vi "ConfigCreateProgram.vi"(9 "Positions":string[][](array[string]), 10 "Microscope":string[][](array[string]), 11 "Single Feed Cycle Refresh Ratio":dbl[](array[numeric])) -> (2 "ProgramPath":path, 3 "ProgramStopped":bool)   [LabVIEW 2018, in "Config.lvlib"]
uses:
  Config.lvlib
  <vilib>/Analysis/baseanly.llb/Mean (DBL).vi
  <vilib>/xml/Load XML File.vi
  <vilib>/xml/Close Reference(Node).vi
  <vilib>/xml/NI_XML.lvlib
  <vilib>/Analysis/NI_AALBase.lvlib
panel:
  out "LoopEndNumber":u16
  out "LoopStartNumber":u16
  in  "error in":errorcluster
  in  "Calc Minimal Acqu time":bool
  out "Minimal Acquisition Time":dbl format="%<%H:%M:%S>t"
  out "Micro Ok?":bool
  in  "Microscope Settings":path
  out "Pos Ok?":bool
  in  "Load Positions":path
  in  "Acquire":bool
  in  "Loop End":bool
  in  "Loop Start":bool
  in  "Incubate":bool
  in  "Change Reagent":bool
  in  "Feed":bool
  in  "Mix":bool
  out "error out":errorcluster
  in  "Program Steps":i32(listbox)
  in  "stop":bool
  in  "Load old Prog":bool
  in  "Clear":bool
  in  "Save":bool
  # "Program Creation"
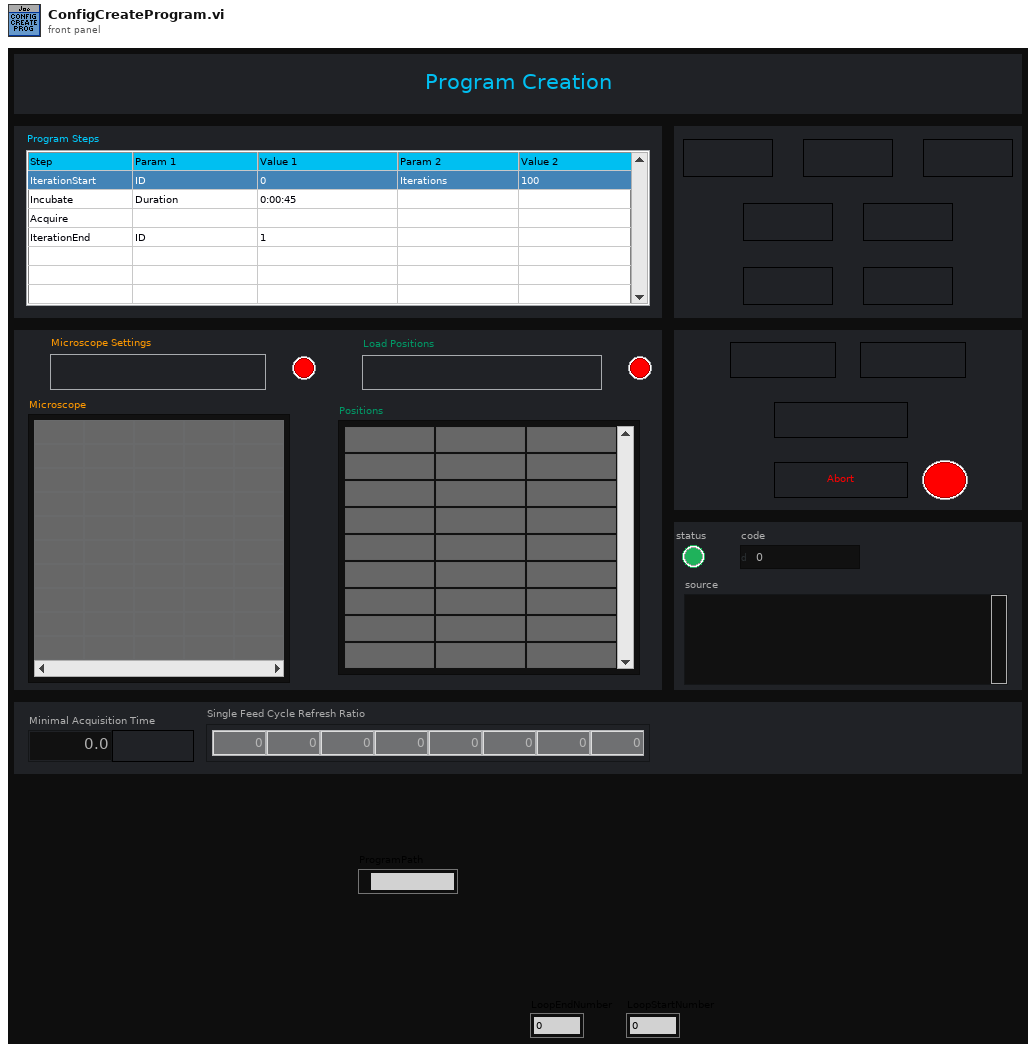
[diagram p1: front panel]
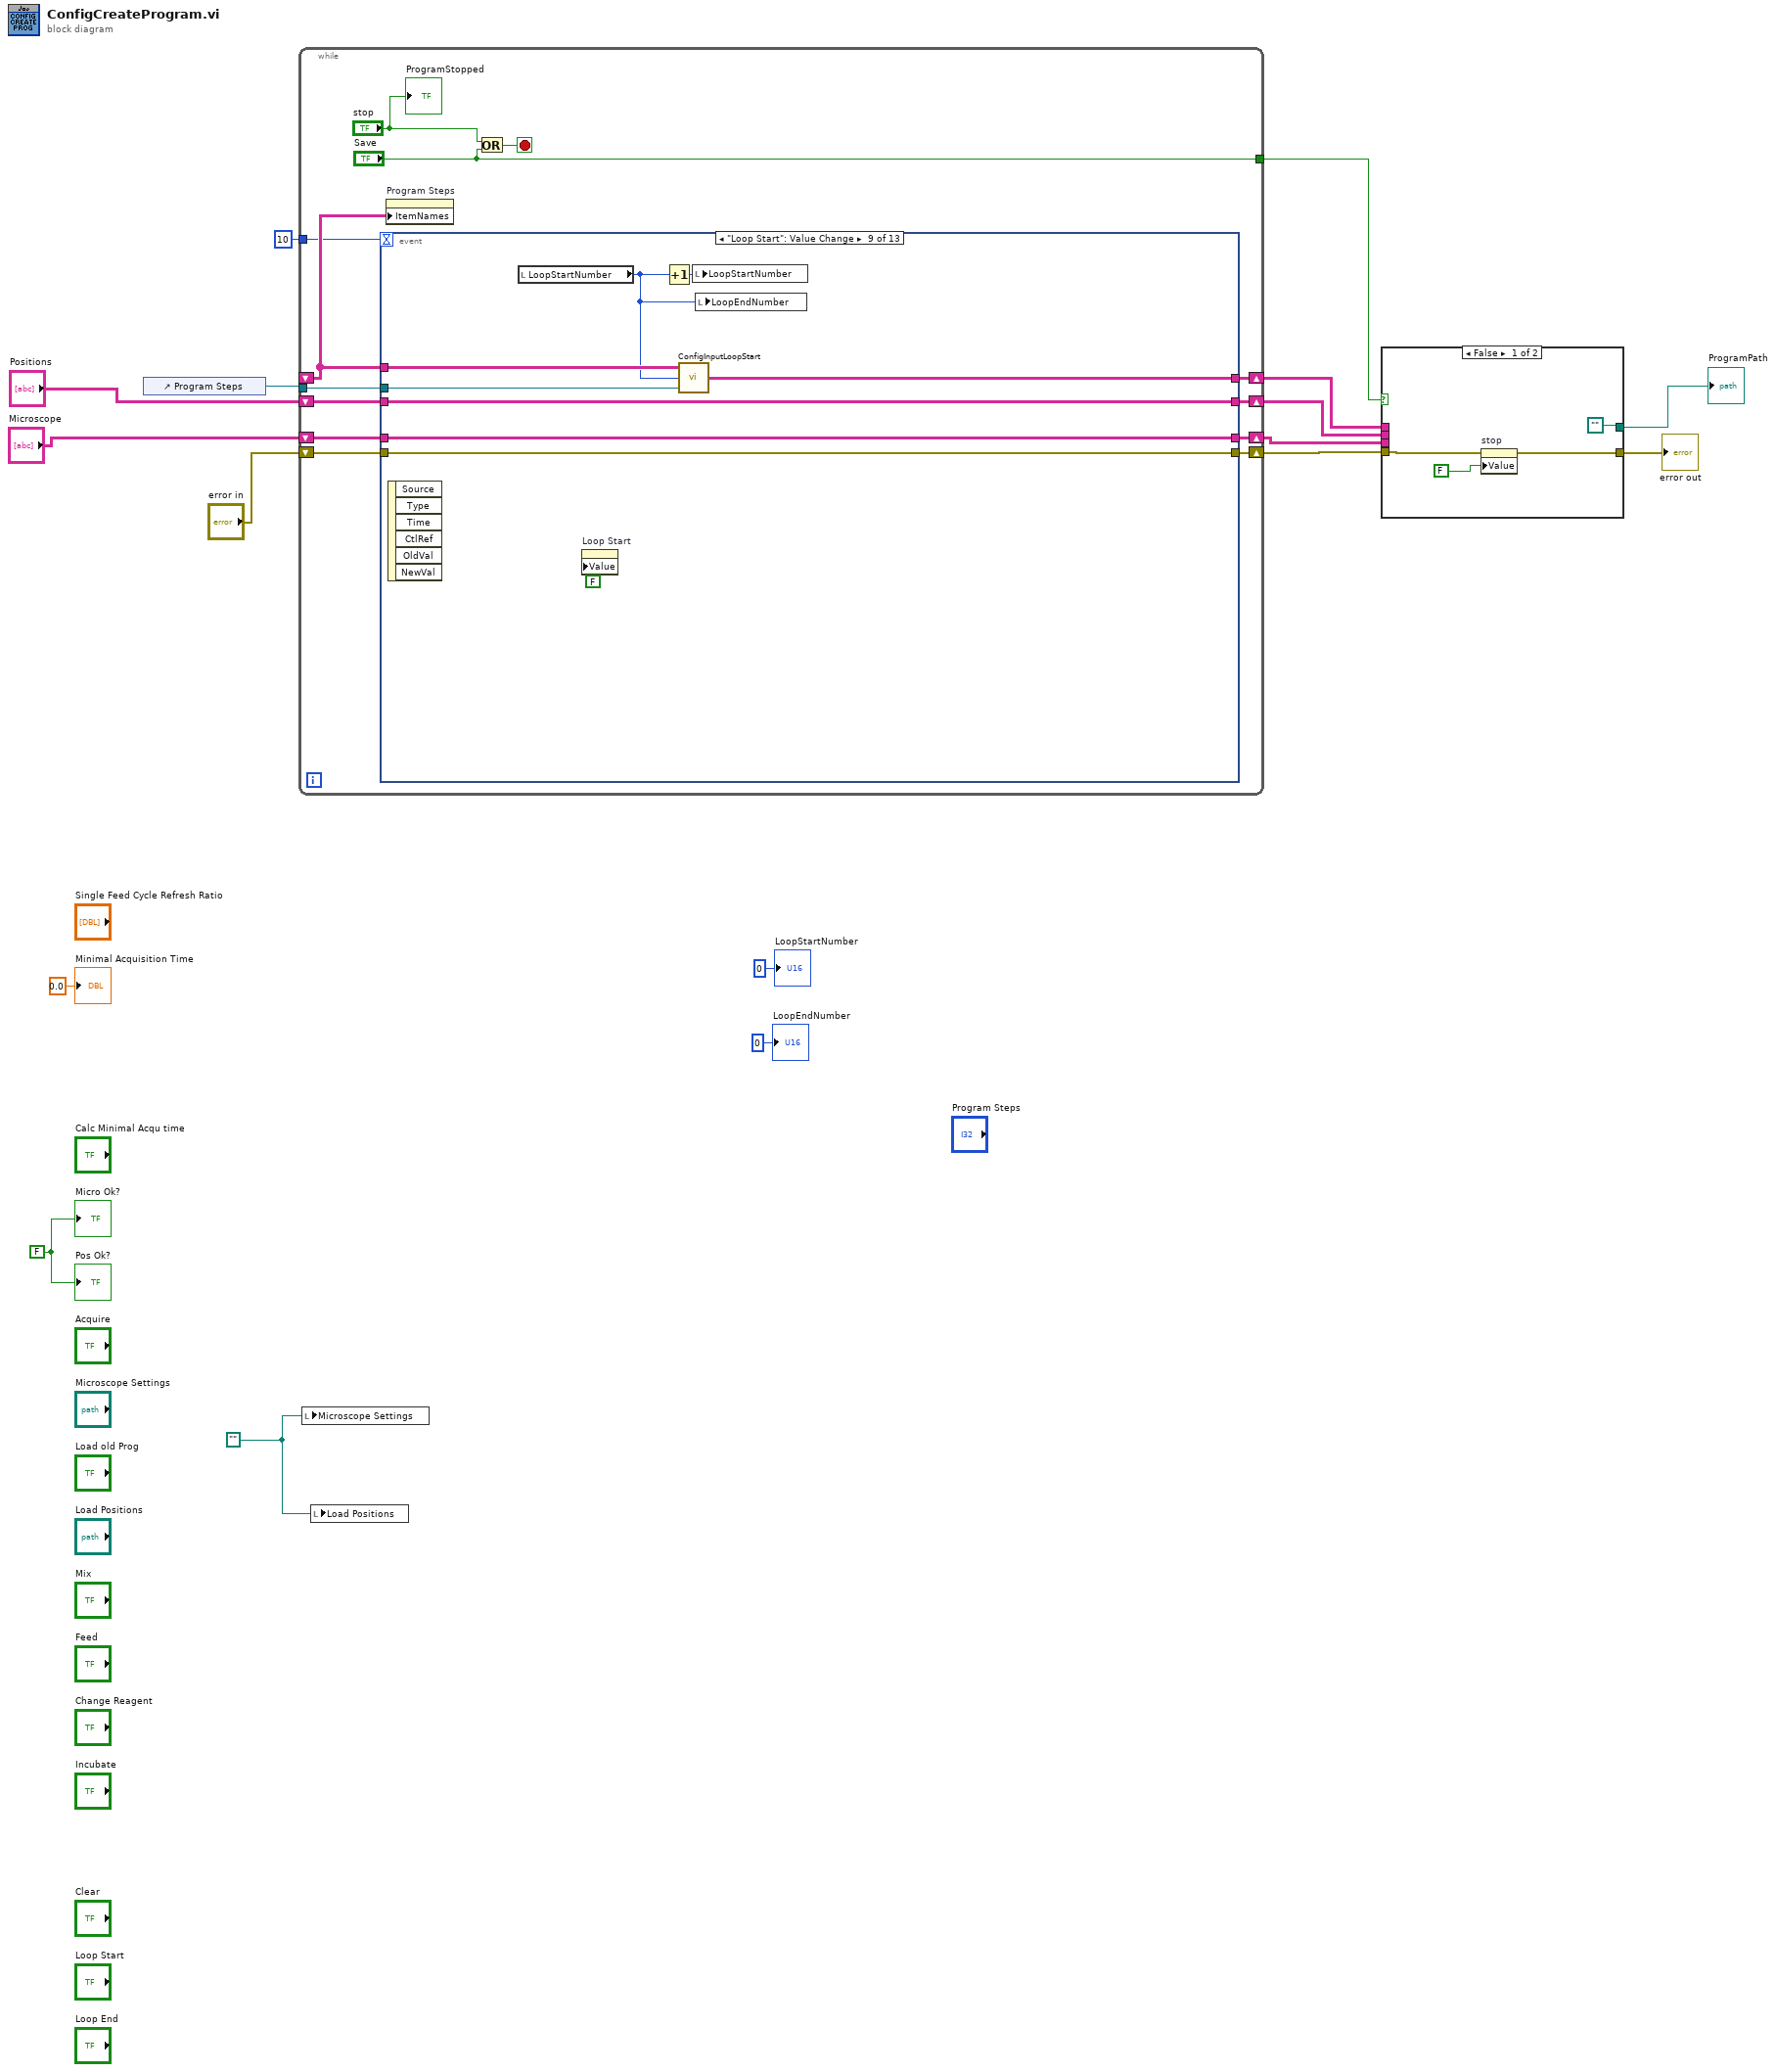
[diagram p0: block diagram]
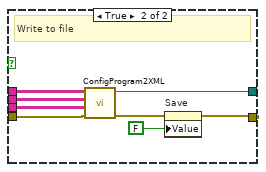
[diagram p2: hidden frame]
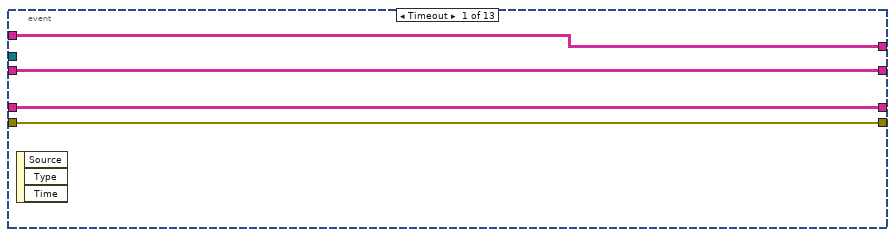
[diagram p3: hidden frame]
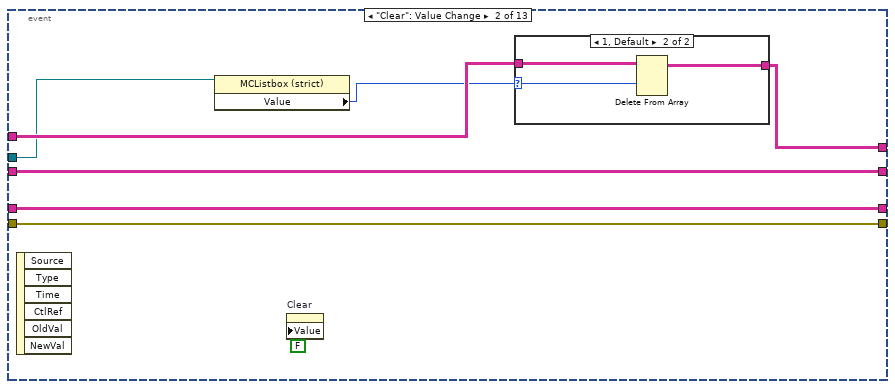
[diagram p4: hidden frame]
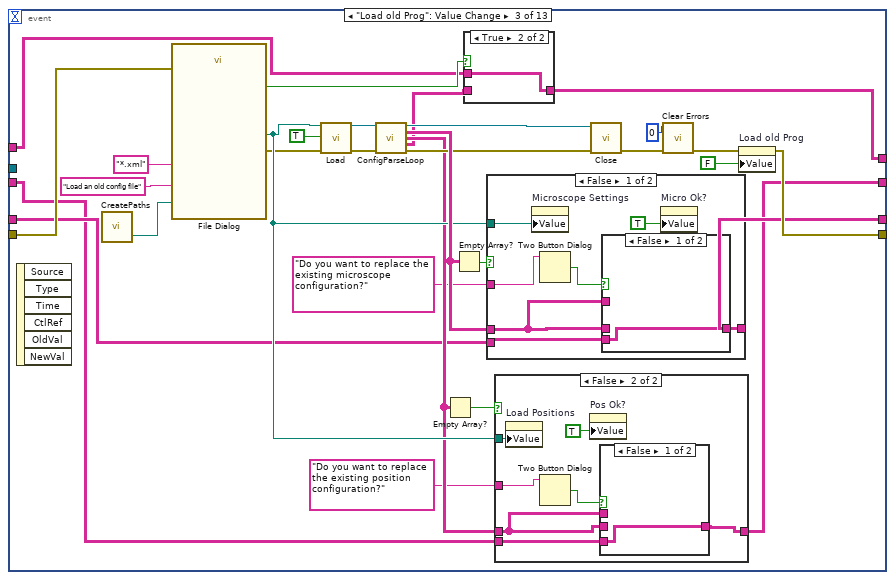
[diagram p6: hidden frame]
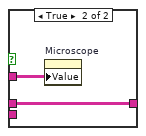
[diagram p8: hidden frame]
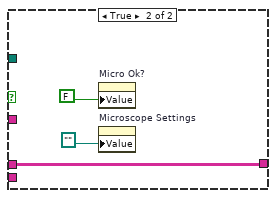
[diagram p9: hidden frame]
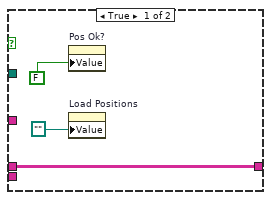
[diagram p10: hidden frame]
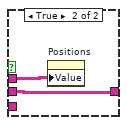
[diagram p11: hidden frame]
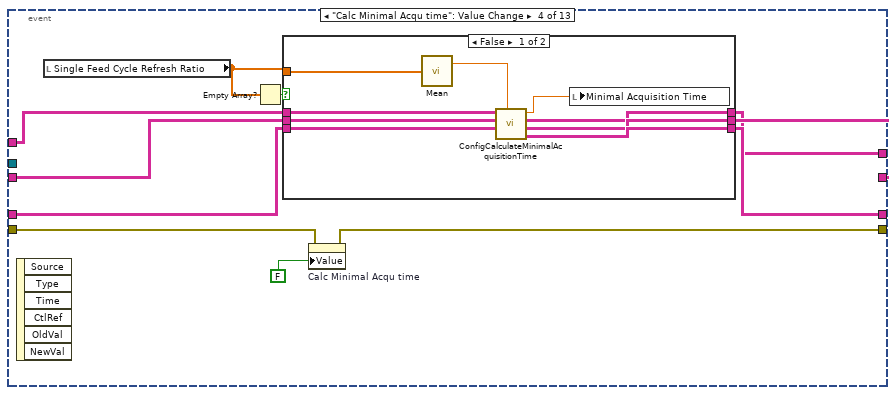
[diagram p12: hidden frame]
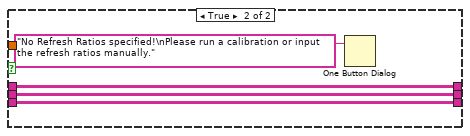
[diagram p13: hidden frame]
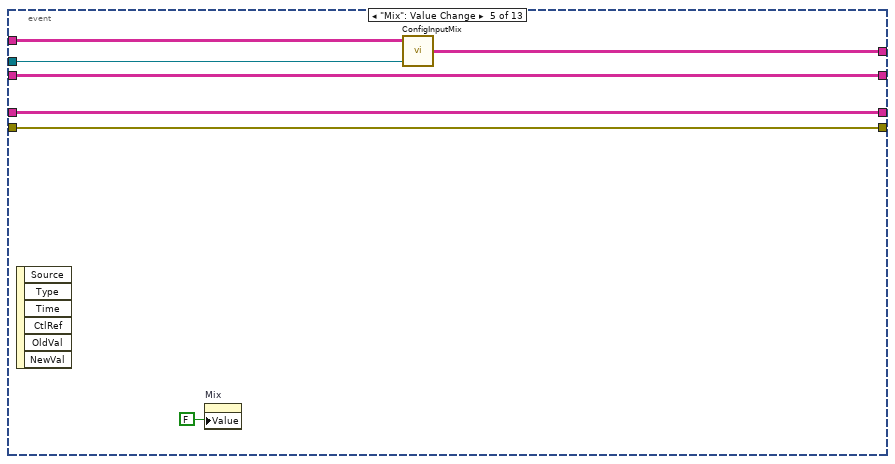
[diagram p14: hidden frame]
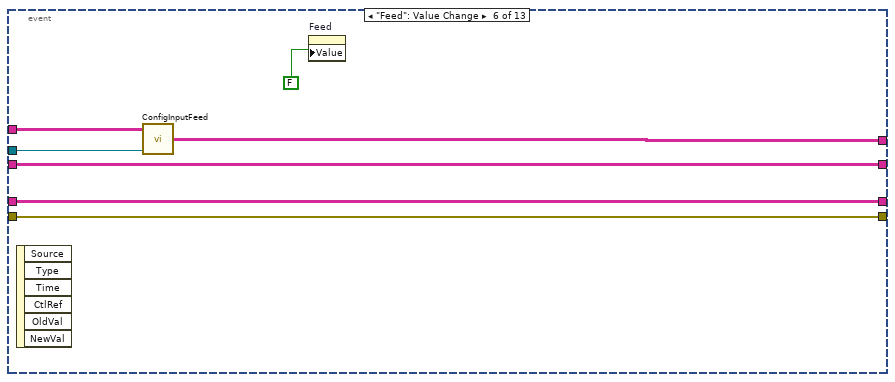
[diagram p15: hidden frame]
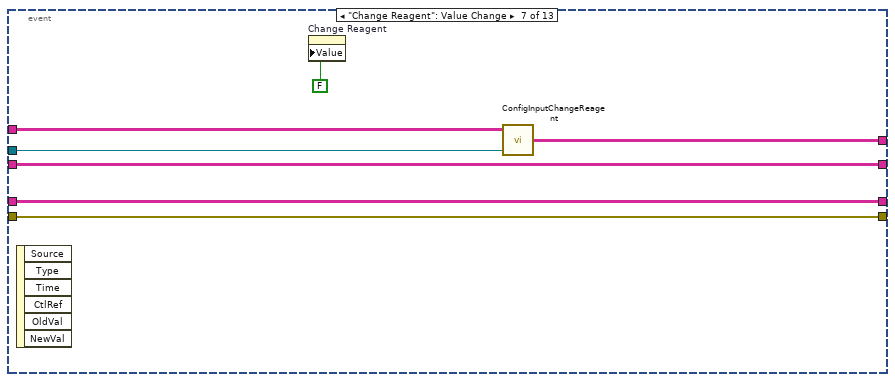
[diagram p16: hidden frame]
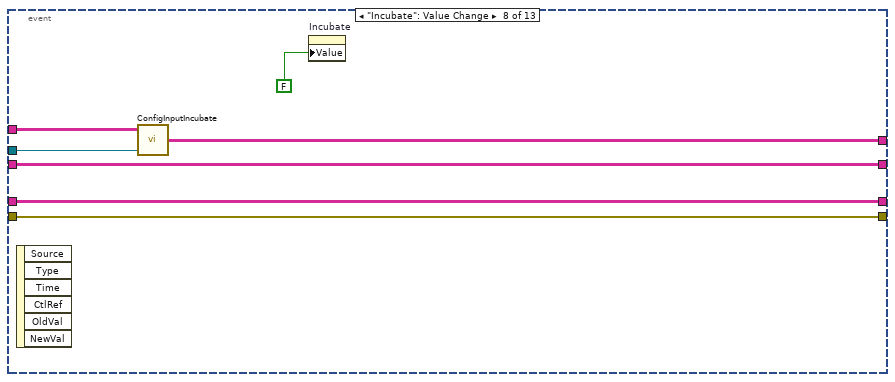
[diagram p17: hidden frame]
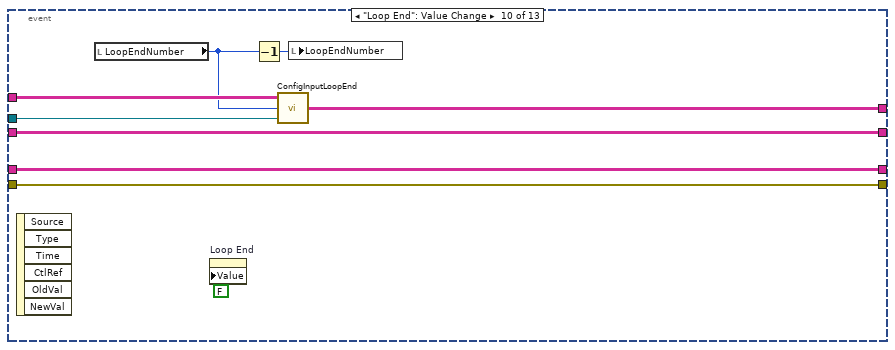
[diagram p18: hidden frame]
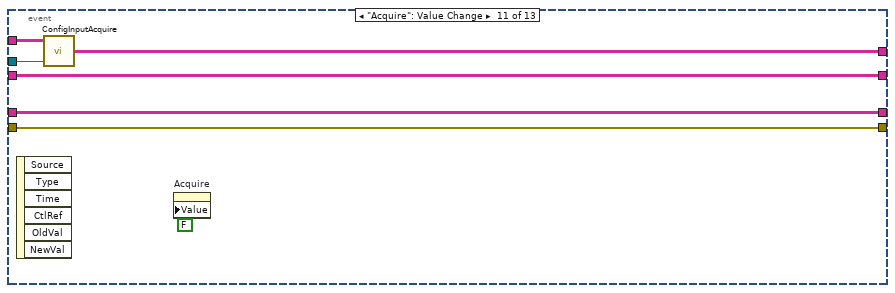
[diagram p19: hidden frame]
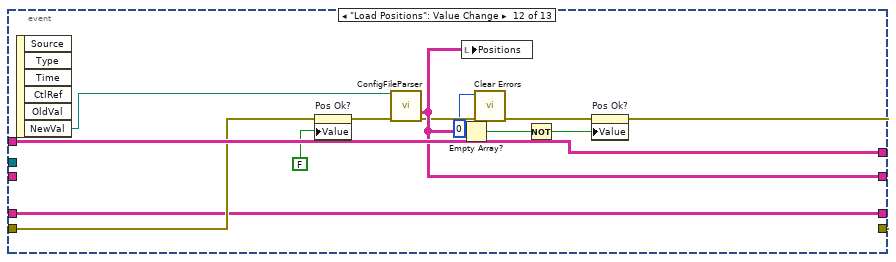
[diagram p20: hidden frame]
diagram:
  w9 = FALSE
  w10 = path ""
  n1 = control-ref of="Program Steps"() -> (w11:refnum<vi>)
  n2 = while {
    shift-right: [w30] -> w16
    shift-left: _ -> [w27]
    shift-right: [w28] -> w14
    shift-left: "error in" -> [w29]
    shift-right: [w24] -> w12
    shift-left: "Positions" -> [w23]
    shift-right: [w25] -> w15
    shift-left: "Microscope" -> [w26]
    tunnel: ["Save"] -> w13
    tunnel: w11 -> [w21]
    tunnel: 10 -> [w20]
    stop <- w22 stop-if-true
    n3 = event shown="[8] \"Loop Start\": Value Change" {
      selector: _ -> [_ _ _ _ _ _ _ _ _ _ _ _ _]
      dyn-events: _ -> [_ _ _ _ _ _ _ _ _ _ _ _ _]
      timeout: w20 -> [_ _ _ _ _ _ _ _ _ _ _ _ _]
      tunnel: w27 -> [w34 w42 w47 w111 w129 w137 w144 w151 w159 w168 w176 w193 w206]
      tunnel: [w34 w37 w48 w106 w130 w135 w142 w149 w156 w166 w174 w193 w206] -> w30
      tunnel: w29 -> [w33 w40 w72 w112 w131 w140 w147 w154 w163 w172 w179 w188 w201]
      tunnel: [w33 w40 w66 w114 w131 w140 w147 w154 w163 w172 w179 w187 w200] -> w28
      tunnel: [w32 w39 w55 w107 w132 w139 w146 w153 w162 w171 w178 w186 w198] -> w24
      tunnel: w26 -> [w31 w38 w52 w109 w133 w138 w145 w152 w161 w170 w177 w185 _]
      tunnel: [w31 w38 w56 w108 w133 w138 w145 w152 w161 w170 w177 w185 w199] -> w25
      tunnel: w23 -> [w32 w39 w51 w110 w132 w139 w146 w153 w162 w171 w178 _ w198]
      tunnel: w21 -> [_ w36 _ _ w128 w136 w143 w150 w158 w167 w175 _ _]
      event Timeout {
        n4 = event-data() -> ()  [unwired: 1 in, 3 out]
      }
      event "Clear": Value Change {
        n5 = event-data() -> ()  [unwired: 1 in, 6 out]
        n6 = property class="MCListbox (strict)"(reference=w36) -> ("Value"=w35:i32)  [unwired: 1 in, 2 out]
        n7 = property on="Clear" class="Bool (strict)"("Value"=FALSE ("Value (Signaling)")) -> ()  [unwired: 2 in, 2 out]
        n8 = case shown="1, Default" w35 {
          selector: w35 -> [_ w44]
          tunnel: [w43 w46] -> w37
          tunnel: w42 -> [w43 w45]
          frame -1 {
          }
          frame 1, Default {
            n9 = Delete From Array(array=w45, index (row)=w44) -> (array with subset deleted=w46:string[][])  [unwired: 2 in, 1 out]
          }
        }
      }
      event "Load old Prog": Value Change {
        w58 = TRUE ("process namespaces (False)")
        n10 = event-data() -> ()  [unwired: 1 in, 6 out]
        n11 = call "CreatePaths.vi"() -> ("ConfigFilesPath"=w59:path)  [unwired: 2 in, 1 out]
        n12 = call "File Dialog"("start path"=w59, "prompt"="Load an old config file", "error in"=w72, "pattern label"="*.xml") -> ("selected path"=w67:path, "cancelled"=w50:bool, "error out"=w63:errorcluster)  [unwired: 8 in, 1 out]
        n13 = call-poly <vilib>:"Load.vi"("path to XML document"=w67, "process namespaces (False)"=w58, "process schema (False)"=w58, "error in (no error)"=w63) -> ("DOM document out"=w71:refnum<k20>, "error out"=w64:errorcluster)  [unwired: 9 in, 1 out]
        n14 = call "ConfigParseLoop.vi"("Root Refnum in"=w71, "error in (no error)"=w64) -> ("Loop Microscope Settings"=w68:string[][], "Position Settings"=w57:string[][], "Program"=w49:string[][], "error out"=w65:errorcluster)  [unwired: 9 in, 1 out]
        n15 = Empty Array?(array=w57) -> (empty?=w70:bool)
        n16 = Empty Array?(array=w68) -> (empty?=w69:bool)
        n17 = case shown="True" w50 {
          tunnel: w49 -> [w76 _]
          tunnel: [w76 w77] -> w48
          tunnel: w47 -> [_ w77]
          frame False {
          }
          frame True {
          }
        }
        n18 = case shown="False" w69 {
          tunnel: w68 -> [w82 w88]
          tunnel: w67 -> [w84 _]
          tunnel: [w81 w88] -> w56
          tunnel: "Do you want to replace the existing microscope configuration?" ("message") -> [w79 _]
          tunnel: w52 -> [w78 _]
          frame False {
            n19 = property on="Microscope Settings" class="Path"("Value"=w84) -> ()  [unwired: 2 in, 2 out]
            n20 = Two Button Dialog(message=w79) -> (T button?=w80:bool)  [unwired: 2 in]
            n21 = case shown="False" w80 {
              tunnel: w82 -> [_ w87]
              tunnel: w82 -> [_ w86]
              tunnel: [w85 w86] -> w81
              tunnel: w78 -> [w85 _]
              frame False {
              }
              frame True {
                n22 = property on="Microscope" class="Arr (strict)"("Value"=w87) -> ()  [unwired: 2 in, 2 out]
              }
            }
            n23 = property on="Micro Ok?" class="Bool (strict)"("Value"=TRUE ("Micro Ok?")) -> ()  [unwired: 2 in, 2 out]
          }
          frame True {
            n24 = property on="Micro Ok?" class="Bool (strict)"("Value"=FALSE ("Micro Ok?")) -> ()  [unwired: 2 in, 2 out]
            n25 = property on="Microscope Settings" class="Path"("Value"=path "") -> ()  [unwired: 2 in, 2 out]
          }
        }
        n26 = case shown="False" w70 {
          tunnel: w57 -> [w91 w96]
          tunnel: w67 -> [_ w100]
          tunnel: [w91 w95] -> w55
          tunnel: "Do you want to replace the existing position configuration?" ("message") -> [_ w97]
          tunnel: w51 -> [_ w94]
          frame True {
            n27 = property on="Pos Ok?" class="Bool (strict)"("Value"=FALSE ("Pos Ok?")) -> ()  [unwired: 2 in, 2 out]
            n28 = property on="Load Positions" class="Path"("Value"=path "") -> ()  [unwired: 2 in, 2 out]
          }
          frame False {
            n29 = property on="Load Positions" class="Path"("Value"=w100) -> ()  [unwired: 2 in, 2 out]
            n30 = Two Button Dialog(message=w97) -> (T button?=w98:bool)  [unwired: 2 in]
            n31 = property on="Pos Ok?" class="Bool (strict)"("Value"=TRUE ("Pos Ok?")) -> ()  [unwired: 2 in, 2 out]
            n32 = case shown="False" w98 {
              tunnel: w96 -> [_ w103]
              tunnel: w96 -> [_ w102]
              tunnel: [w101 w102] -> w95
              tunnel: w94 -> [w101 _]
              frame False {
              }
              frame True {
                n33 = property on="Positions" class="Arr (strict)"("Value"=w103) -> ()  [unwired: 2 in, 2 out]
              }
            }
          }
        }
        n34 = call-poly <vilib>:"Close.vi"("error in (no error)"=w65, "node"=w71) -> ("error out"=w61:errorcluster)  [unwired: 7 in]
        n35 = call <vilib>:"Clear Errors.vi"("error in (no error)"=w61, "specific error code to clear (0: all)"=0) -> ("error out"=w60:errorcluster)  [unwired: 4 in, 1 out]
        n36 = property on="Load old Prog" class="Bool (strict)"(error in=w60, "Value"=FALSE ("Value (Signaling)")) -> (error out=w66:errorcluster)  [unwired: 1 in, 1 out]
      }
      event "Calc Minimal Acqu time": Value Change {
        n37 = event-data() -> ()  [unwired: 1 in, 6 out]
        n38 = local read "Single Feed Cycle Refresh Ratio"() -> (w105:dbl[])
        n39 = Empty Array?(array=w105) -> (empty?=w104:bool)
        n40 = case shown="False" w104 {
          tunnel: w111 -> [w123 w127]
          tunnel: w110 -> [w122 w126]
          tunnel: w109 -> [w121 w125]
          tunnel: [w120 w125] -> w108
          tunnel: [w119 w126] -> w107
          tunnel: [w118 w127] -> w106
          tunnel: w105 -> [w116 _]
          frame False {
            n41 = call-poly <vilib>:"Mean.vi"("X"=w116) -> ("mean"=w117:dbl)  [unwired: 1 out]
            n42 = call "ConfigCalculateMinimalAcquisitionTime.vi"("Single Feed Cycle Refresh Ratio"=w117, "Loop Microscope Settings"=w121, "Positions"=w122, "Program"=w123) -> ("Microscope Out"=w120:string[][], "Positions out"=w119:string[][], "Program out"=w118:string[][], "Minimal Acquisition Time"=w115:dbl)  [unwired: 4 in]
            n43 = local write "Minimal Acquisition Time"(w115) -> ()
          }
          frame True {
            n44 = One Button Dialog(message="No Refresh Ratios specified!\nPlease run a calibration or input the refresh ratios manually.") -> ()  [unwired: 1 in, 1 out]
          }
        }
        n45 = property on="Calc Minimal Acqu time" class="Bool (strict)"(error in=w112, "Value"=FALSE ("Calc Minimal Acqu time")) -> (error out=w114:errorcluster)  [unwired: 1 in, 1 out]
      }
      event "Mix": Value Change {
        n46 = event-data() -> ()  [unwired: 1 in, 6 out]
        n47 = property on="Mix" class="Bool (strict)"("Value"=FALSE ("Value (Signaling)")) -> ()  [unwired: 2 in, 2 out]
        n48 = call "ConfigInputMix.vi"("MulticolumnListbox in"=w128, "ItemNames in"=w129) -> ("ItemNames out"=w130:string[][])  [unwired: 1 in]
      }
      event "Feed": Value Change {
        n49 = event-data() -> ()  [unwired: 1 in, 6 out]
        n50 = call "ConfigInputFeed.vi"("MulticolumnListbox in"=w136, "ItemNames in"=w137) -> ("ItemNames out"=w135:string[][])  [unwired: 1 in]
        n51 = property on="Feed" class="Bool (strict)"("Value"=FALSE ("Value (Signaling)")) -> ()  [unwired: 2 in, 2 out]
      }
      event "Change Reagent": Value Change {
        n52 = event-data() -> ()  [unwired: 1 in, 6 out]
        n53 = property on="Change Reagent" class="Bool (strict)"("Value"=FALSE ("Value (Signaling)")) -> ()  [unwired: 2 in, 2 out]
        n54 = call "ConfigInputChangeReagent.vi"("MulticolumnListbox in"=w143, "ItemNames in"=w144) -> ("ItemNames out"=w142:string[][])  [unwired: 1 in]
      }
      event "Incubate": Value Change {
        n55 = event-data() -> ()  [unwired: 1 in, 6 out]
        n56 = call "ConfigInputIncubate.vi"("MulticolumnListbox in"=w150, "ItemNames in"=w151) -> ("ItemNames out"=w149:string[][])  [unwired: 1 in]
        n57 = property on="Incubate" class="Bool (strict)"("Value"=FALSE ("Value (Signaling)")) -> ()  [unwired: 2 in, 2 out]
      }
      event "Loop Start": Value Change {
        n58 = event-data() -> ()  [unwired: 1 in, 6 out]
        n59 = local read "LoopStartNumber"() -> (w157:u16)
        n60 = property on="Loop Start" class="Bool (strict)"("Value"=FALSE ("Value (Signaling)")) -> ()  [unwired: 2 in, 2 out]
        n61 = Increment(x=w157) -> (x+1=w160:u16)
        n62 = call "ConfigInputLoopStart.vi"("MulticolumnListbox in"=w158, "ID"=w157, "ItemNames in"=w159) -> ("ItemNames out"=w156:string[][])
        n63 = local write "LoopStartNumber"(w160) -> ()
        n64 = local write "LoopEndNumber"(w157) -> ()
      }
      event "Loop End": Value Change {
        n65 = event-data() -> ()  [unwired: 1 in, 6 out]
        n66 = local read "LoopEndNumber"() -> (w165:u16)
        n67 = property on="Loop End" class="Bool (strict)"("Value"=FALSE ("Value (Signaling)")) -> ()  [unwired: 2 in, 2 out]
        n68 = Decrement(x=w165) -> (x-1=w169:u16)
        n69 = call "ConfigInputLoopEnd.vi"("MulticolumnListbox in"=w167, "ID"=w165, "ItemNames in"=w168) -> ("ItemNames out"=w166:string[][])
        n70 = local write "LoopEndNumber"(w169) -> ()
      }
      event "Acquire": Value Change {
        n71 = event-data() -> ()  [unwired: 1 in, 6 out]
        n72 = call "ConfigInputAcquire.vi"("MulticolumnListbox in"=w175, "ItemNames in"=w176) -> ("ItemNames out"=w174:string[][])  [unwired: 1 in]
        n73 = property on="Acquire" class="Bool (strict)"("Value"=FALSE ("Value (Signaling)")) -> ()  [unwired: 2 in, 2 out]
      }
      event "Load Positions": Value Change {
        n74 = event-data() -> ("NewVal"=w192:path)  [unwired: 1 in, 5 out]
        n75 = property on="Pos Ok?" class="Bool (strict)"(error in=w188, "Value"=FALSE) -> (error out=w183:errorcluster)  [unwired: 1 in, 1 out]
        n76 = call "ConfigFileParser.vi"("Path"=w192, "error in"=w183) -> ("Positions"=w186:string[][], "error out"=w184:errorcluster)  [unwired: 8 in, 4 out]
        n77 = Empty Array?(array=w186) -> (empty?=w190:bool)
        n78 = local write "Positions"(w186) -> ()
        n79 = call <vilib>:"Clear Errors.vi"("error in (no error)"=w184, "specific error code to clear (0: all)"=0) -> ("error out"=w182:errorcluster)  [unwired: 4 in, 1 out]
        n80 = Not(x=w190) -> (.not. x?=w191:bool)
        n81 = property on="Pos Ok?" class="Bool (strict)"(error in=w182, "Value"=w191) -> (error out=w187:errorcluster)  [unwired: 1 in, 1 out]
      }
      event "Microscope Settings": Value Change {
        n82 = event-data() -> ("NewVal"=w205:path)  [unwired: 1 in, 5 out]
        n83 = property on="Micro Ok?" class="Bool (strict)"(error in=w201, "Value"=FALSE) -> (error out=w194:errorcluster)  [unwired: 1 in, 1 out]
        n84 = call "ConfigFileParser.vi"("Path"=w205, "error in"=w194) -> ("Loop Microscope Settings"=w199:string[][], "error out"=w195:errorcluster)  [unwired: 8 in, 4 out]
        n85 = Empty Array?(array=w199) -> (empty?=w203:bool)
        n86 = call <vilib>:"Clear Errors.vi"("error in (no error)"=w195, "specific error code to clear (0: all)"=0) -> ("error out"=w196:errorcluster)  [unwired: 4 in, 1 out]
        n87 = Not(x=w203) -> (.not. x?=w204:bool)
        n88 = property on="Micro Ok?" class="Bool (strict)"(error in=w196, "Value"=w204) -> (error out=w200:errorcluster)  [unwired: 1 in, 1 out]
        n89 = local write "Microscope"(w199) -> ()
      }
    }
    n90 = property on="Program Steps" class="MCListbox (strict)"("ItemNames"=w27) -> ()  [unwired: 2 in, 2 out]
    n91 = Or(x="stop", y="Save") -> (x .or. y?=w22:bool)
    "ProgramStopped" <- "stop"
  }
  n92 = local write "Microscope Settings"(w10) -> ()
  n93 = local write "Load Positions"(w10) -> ()
  n94 = case shown="False" w13 {
    tunnel: [w208 w218] -> w17
    tunnel: w16 -> [_ w215]
    tunnel: w15 -> [_ w212]
    tunnel: w14 -> [w209 w214]
    tunnel: w12 -> [_ w213]
    tunnel: [path "" w211] -> w3
    frame False {
      n95 = property on="stop" class="Bool (strict)"(error in=w209, "Value"=FALSE ("stop")) -> (error out=w208:errorcluster)  [unwired: 1 in, 1 out]
    }
    frame True {
      # "Write to file"
      n96 = call "ConfigProgram2XML.vi"("error in (no error)"=w214, "Microscope"=w212, "Positions"=w213, "Program"=w215) -> ("error out"=w217:errorcluster, "ProgramPath"=w211:path)  [unwired: 6 in]
      n97 = property on="Save" class="Bool (strict)"(error in=w217, "Value"=FALSE ("Save")) -> (error out=w218:errorcluster)  [unwired: 1 in, 1 out]
    }
  }
  "error out" <- w17
  "ProgramPath" <- w3
  "Pos Ok?" <- w9
  "Micro Ok?" <- w9
  "Minimal Acquisition Time" <- 0.0 ("Minimal Acquisition Time")
  "LoopStartNumber" <- u16 0 ("LoopNumber")
  "LoopEndNumber" <- u16 0 ("LoopEndNumber")
